vi "SimpleElapsedMissionClock.vi"() -> ()   [LabVIEW 2010]
panel:
  out "x-y":dbl
  out "current time 2":timestamp
  out "current time":timestamp
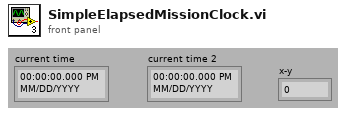
[diagram p1: front panel]
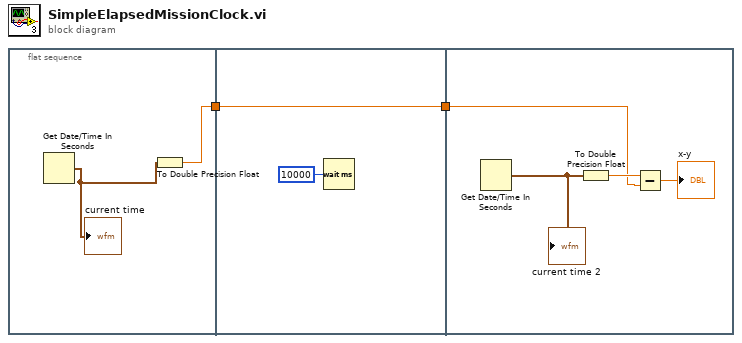
[diagram p0: block diagram]
diagram:
  n1 = flat-sequence {
    tunnel: [w3] -> w1
    tunnel: [w5] -> w2
    tunnel: w1 -> [w5]
    tunnel: w2 -> [w8]
    frame #0 {
      n2 = Get Date/Time In Seconds() -> (seconds since 1Jan1904=w4:timestamp)
      "current time" <- w4
      n3 = To Double Precision Float(number=w4) -> (double precision float=w3:dbl)
    }
    frame #1 {
      n4 = Wait (ms)(milliseconds to wait=u32 10000) -> ()  [unwired: 1 out]
    }
    frame #2 {
      n5 = Get Date/Time In Seconds() -> (seconds since 1Jan1904=w10:timestamp)
      "current time 2" <- w10
      n6 = To Double Precision Float(number=w10) -> (double precision float=w9:dbl)
      n7 = Subtract(x=w9, y=w8) -> (x-y=→"x-y":dbl)
    }
  }
